vi "RateLimiter.vi"(7 "Reset":bool, 10 "Max dx/dt":dbl=1.0, 11 "Input":dbl(slide) scale=-10.0..10.0) -> (3 "Output":dbl)   [LabVIEW 2017]
doc: "The output tries to reach the input but can only change at a rate of Max dx/dt"
panel:
  # "r"
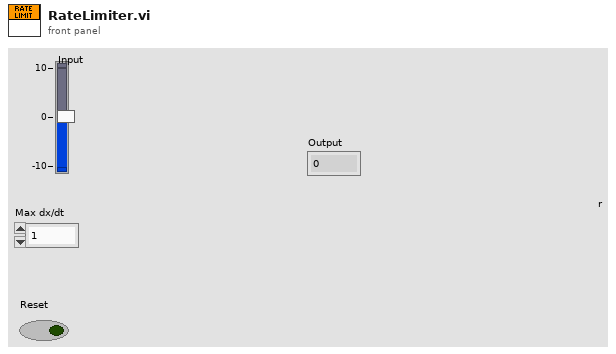
[diagram p1: front panel]
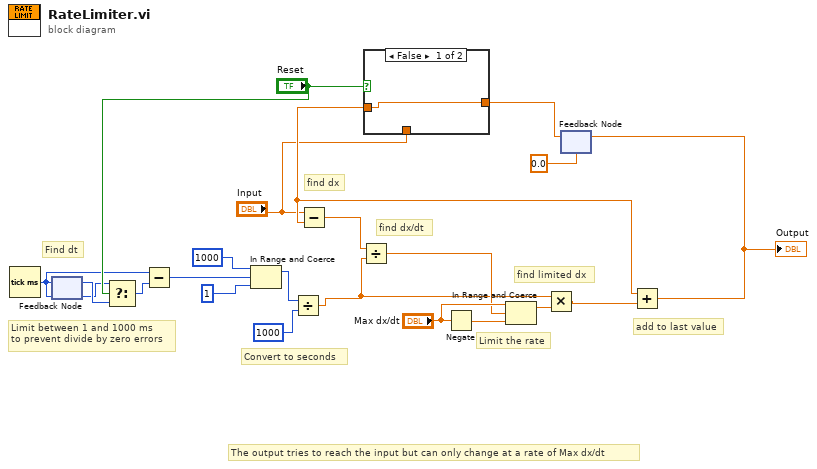
[diagram p0: block diagram]
diagram:
  # "The output tries to reach the input but can only change at a rate of Max dx/dt"
  # "Convert to seconds"
  # "find limited dx"
  # "add to last value"
  # "Limit the rate"
  # "find dx/dt"
  # "find dx"
  # "Limit between 1 and 1000 ms\nto prevent divide by zero errors"
  # "Find dt"
  n1 = Tick Count (ms)() -> (millisecond timer value=w2:u32)
  n2 = feedback-in #1(w2) -> ()
  n3 = feedback #1(w2) -> (w4:u32)
  n4 = Select(t=w2, s="Reset", f=w4) -> (s? t:f=w3:u32)
  n5 = Subtract(x=w2, y=w3) -> (x-y=w11:u32)
  n6 = In Range and Coerce(upper limit=u32 1000, x=w11, lower limit=u32 1) -> (coerced(x)=w8:u32)  [unwired: 1 out]
  n7 = Divide(x=w8, y=u32 1000) -> (x/y=w12:dbl)
  n8 = Negate(x="Max dx/dt") -> (-x=w20:dbl)
  n9 = feedback #2(0.0 ("x-y")) -> (w7:dbl)
  n10 = case shown="False" "Reset" {
    tunnel: w7 -> [w22 _]
    tunnel: [w22 w23] -> w6
    tunnel: "Input" -> [_ w23]
    frame False {
    }
    frame True {
    }
  }
  n11 = Subtract(x="Input", y=w6) -> (x-y=w17:dbl)
  n12 = Divide(x=w17, y=w12) -> (x/y=w16:dbl)
  n13 = In Range and Coerce(upper limit="Max dx/dt", x=w16, lower limit=w20) -> (coerced(x)=w14:dbl)  [unwired: 1 out]
  n14 = Multiply(x=w12, y=w14) -> (x*y=w13:dbl)
  n15 = Add(x=w6, y=w13) -> (x+y=w15:dbl)
  "Output" <- w15
  n16 = feedback-in #2(w15) -> ()
